vi "Line Size (pretty print).vi"() -> (3 "Line Size":i32)   [LabVIEW 2019, in "JSONtext.lvlib"]
uses:
  JSONtext.lvlib
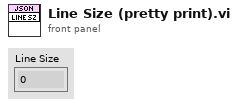
[diagram p1: front panel]
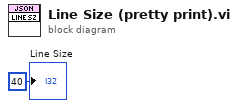
[diagram p0: block diagram]
diagram:
  "Line Size" <- 40 ("y")
